vi "Close.vi"(8 "error in (no error)":errorcluster, 11 "reference in":refnum<class "GarageDoor.lvclass">) -> (0 "error out":errorcluster, 3 "reference out":refnum<class "GarageDoor.lvclass">)   [LabVIEW 2012, in "GarageDoor.lvclass"]
uses:
  GarageDoor.lvclass
  <userlib>/_LabVIEWCommon/LcDialogs/LcDialog_AutoSizeDialog_Font.ctl
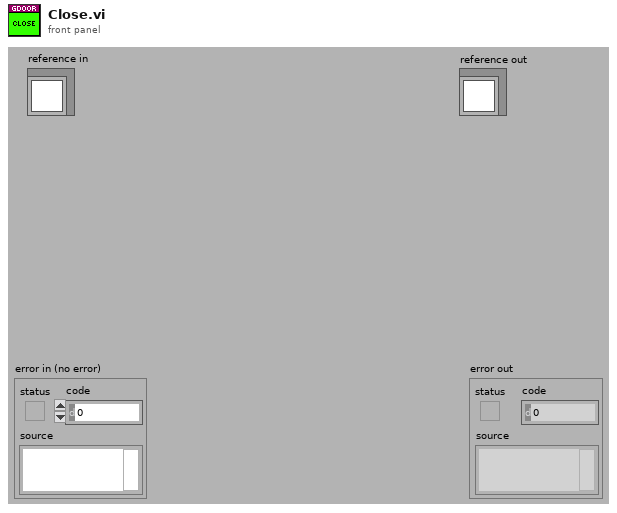
[diagram p1: front panel]
types:
  T1 = typedef "LcDialog_AutoSizeDialog_Font.ctl" = cluster{"Size":u32, "Bold":bool, "Color":u32}
  T2 = typedef "GarageDoor.lvclass/ObjectAttributes.ctl" = cluster{"None":bool}
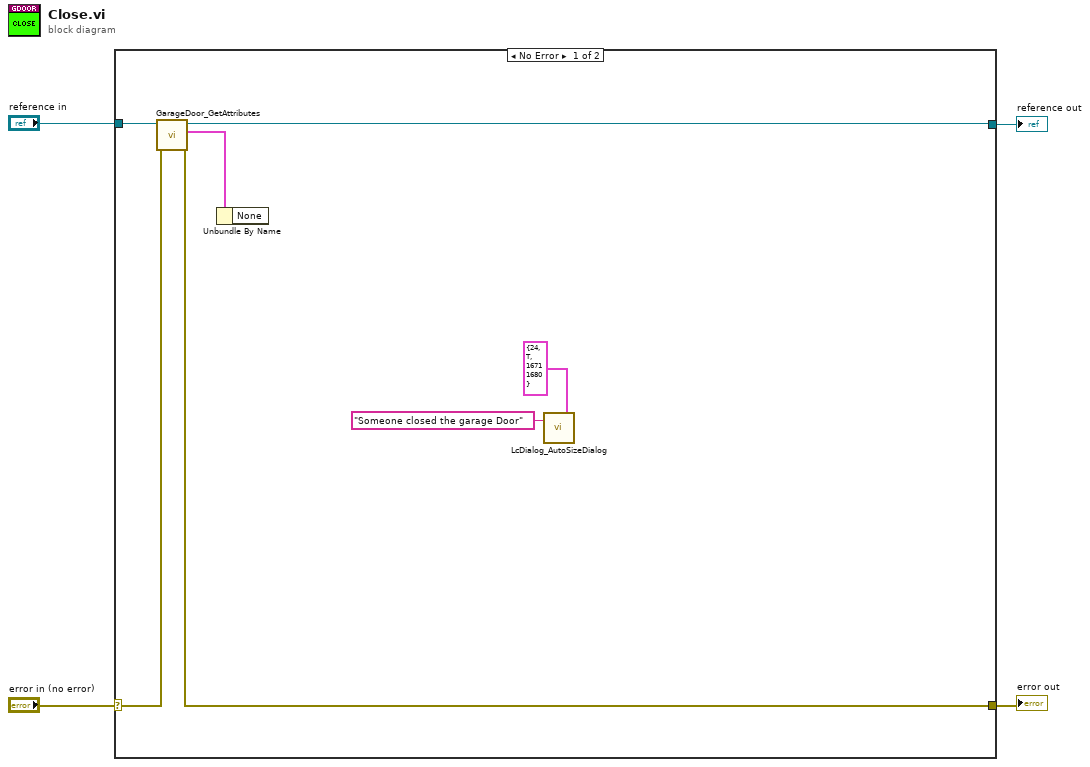
[diagram p0: block diagram]
diagram:
  n1 = case shown="No Error" "error in (no error)" {
    selector: "error in (no error)" -> [w10 w13]
    tunnel: [w7 w13] -> w3
    tunnel: [w8 w12] -> w1
    tunnel: "reference in" -> [w11 w12]
    frame No Error {
      n2 = call "GarageDoor_GetAttributes.vi"("error in (no error)"=w10, "reference in"=w11) -> ("error out"=w7:errorcluster, "Data"=w9:T2, "reference out"=w8:refnum<class "GarageDoor.lvclass">)  [unwired: 6 in, 1 out]
      n3 = Unbundle By Name(w9) -> ()  [unwired: 1 out]
      n4 = call <userlib>:"LcDialog_AutoSizeDialog.vi"("TextIn"="Someone closed the garage Door", "FontSettings"=T1 {"Size"=24, "Bold"=TRUE, "Color"=16711680}) -> ()  [unwired: 13 in, 5 out]
    }
    frame Error {
    }
  }
  "error out" <- w3
  "reference out" <- w1
